vi "Read-all-variables.vi"(8 "error in (no error)":errorcluster, 11 "Storage params. ref. in":refnum<data-value>) -> (0 "error out":errorcluster, 2 "Storage vars.":T1, 3 "Storage params. ref.":refnum<data-value>)   [LabVIEW 2013, in "CameraVision.lvlib" / "CV-Storage.lvclass"]
uses:
  CV-Storage.lvclass
  Storage-variables.ctl
  UI/Module-states.ctl
  CV-Storage.lvclass/CV-Storage.ctl
  UI/CV-UI.lvclass
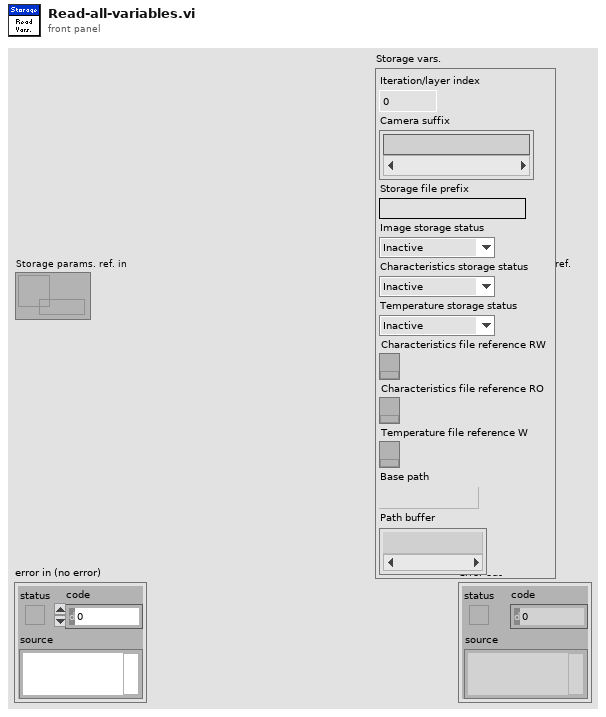
[diagram p1: front panel]
types:
  T1 = typedef "CameraVision.lvlib/CV-Storage.lvclass/Storage-variables.ctl" = cluster{"Iteration/layer index":u16, "Camera suffix":string[], "Storage file prefix":string, "Image storage status":T2, "Characteristics storage status":T2, "Temperature storage status":T2, "Characteristics file reference RW":refnum<k34>, "Characteristics file reference RO":refnum<k34>, "Temperature file reference W":refnum<k34>, "Base path":path, "Path buffer":path[]}
  T2 = typedef "CameraVision.lvlib/CV-UI.lvclass/Module-states.ctl" = enum16{"Inactive", "Active", "Data-loss", "Error", "Simulation", "Synchronizing", "Initialized", "Released"}
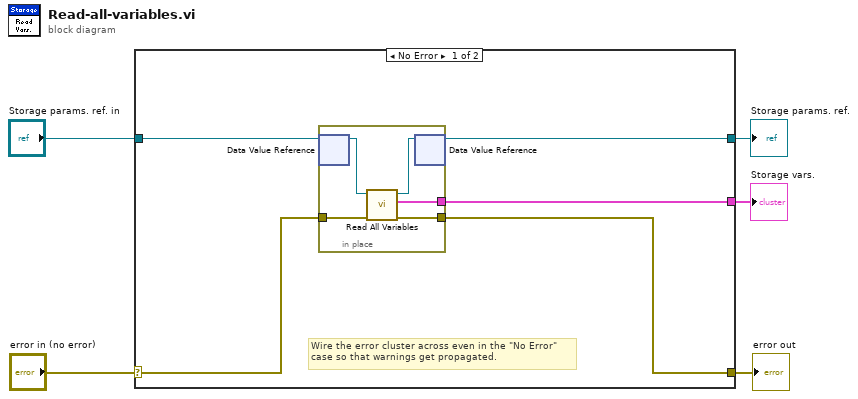
[diagram p0: block diagram]
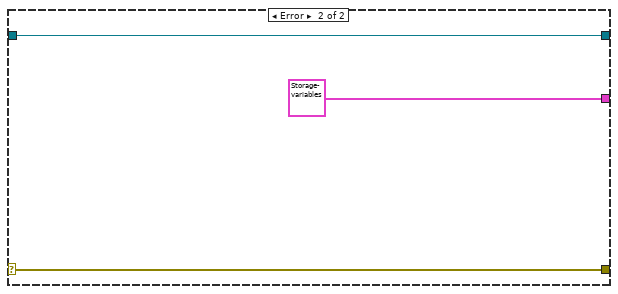
[diagram p2: hidden frame]
diagram:
  n1 = case shown="No Error" "error in (no error)" {
    selector: "error in (no error)" -> [w8 w18]
    tunnel: [w10 w18] -> w4
    tunnel: "Storage params. ref. in" -> [w7 w16]
    tunnel: [w9 T1 {"Iteration/layer index"=0, "Camera suffix"=[], "Storage file prefix"="", "Image storage status"=enum."Inactive", "Characteristics storage status"=enum."Inactive", "Temperature storage status"=enum."Inactive", "Characteristics file reference RW"=refnum, "Characteristics file reference RO"=refnum, "Temperature file reference W"=refnum, "Base path"=path "", "Path buffer"=[]} ("Storage vars.")] -> w2
    tunnel: [w6 w16] -> w1
    frame No Error {
      # "Wire the error cluster across even in the \"No Error\"\ncase so that warnings get propagated."
      n2 = in-place {
        in-place-border: [w15] -> w10
        in-place-border: [w14] -> w9
        in-place-border: w8 -> [w13]
        n3 = in-place-dvr #1(w7) -> (w11:refnum<class "CV-Storage.lvclass">)  [unwired: 1 out]
        n4 = call "Read All Variables.vi"("error in (no error)"=w13, "Storage params in"=w11) -> ("error out"=w15:errorcluster, "Storage vars."=w14:T1, "Storage params out"=w12:refnum<class "CV-Storage.lvclass">)  [unwired: 7 in]
        n5 = in-place-dvr #1(w12) -> (w6:refnum<data-value>)  [unwired: 1 out]
      }
    }
    frame Error {
    }
  }
  "error out" <- w4
  "Storage params. ref." <- w1
  "Storage vars." <- w2
